vi "Read Buffer Statistic.vi"(7 "Statistic (0:Min)":i32(ring) items=["Min", "Max", "Mean", "Standard Deviation", "Peak-to-Peak"], 8 "error in (no error)":errorcluster, 10 "Instrument Model":i32(ring) items=["MODEL 6517B", "MODEL 6517A", "MODEL 6514"], 11 "VISA resource name":refnum<visa-resource-name>) -> (0 "error out":errorcluster, 2 "Statistic Value":dbl, 3 "VISA resource name out":refnum<visa-resource-name>)   [LabVIEW 2016, in "Keithley 6517.lvlib"]
doc: "Reads the specified statistic of the buffer."
uses:
  <instrlib>/Keithley 6517/Keithley 6517.lvlib
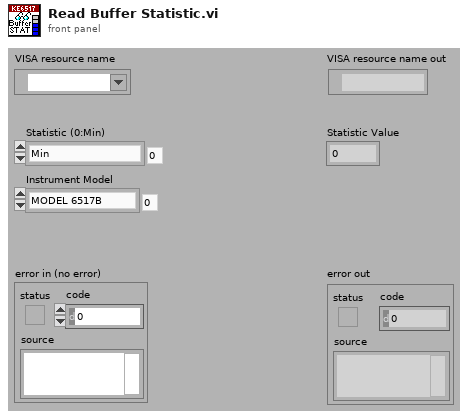
[diagram p1: front panel]
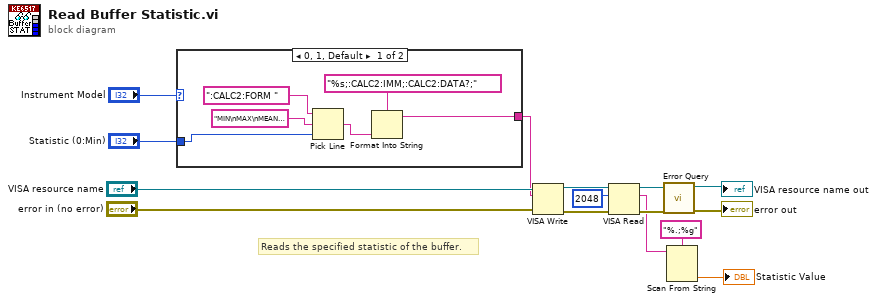
[diagram p0: block diagram]
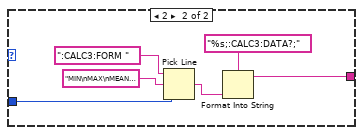
[diagram p2: hidden frame]
diagram:
  # "Reads the specified statistic of the buffer."
  n1 = case shown="0, 1, Default" "Instrument Model" {
    tunnel: "Statistic (0:Min)" -> [w16 w25]
    tunnel: [w17 w22] -> w1
    frame 0, 1, Default {
      n2 = Pick Line(string ("")=":CALC2:FORM ", multi-line string="MIN\nMAX\nMEAN\nSDEV\nPKPK", line index=w16) -> (output string=w19:string)
      n3 = Format Into String(format string="%s;:CALC2:IMM;:CALC2:DATA?;", w19) -> (resulting string=w17:string)  [unwired: 2 in, 1 out]
    }
    frame 2 {
      n4 = Pick Line(string ("")=":CALC3:FORM ", multi-line string="MIN\nMAX\nMEAN\nSDEV\nPKPK", line index=w25) -> (output string=w24:string)
      n5 = Format Into String(format string="%s;:CALC3:DATA?;", w24) -> (resulting string=w22:string)  [unwired: 2 in, 1 out]
    }
  }
  n6 = VISA Write(VISA resource name="VISA resource name", write buffer=w1, error in (no error)="error in (no error)") -> (VISA resource name out=w14:refnum<visa-resource-name>, error out=w15:errorcluster)  [unwired: 1 out]
  n7 = VISA Read(VISA resource name=w14, byte count=u32 2048, error in (no error)=w15) -> (VISA resource name out=w10:refnum<visa-resource-name>, read buffer=w6:string, error out=w11:errorcluster)  [unwired: 1 out]
  n8 = call <instrlib>:"Error Query.vi"("error in (no error)"=w11, "VISA resource name"=w10) -> ("error out"=→"error out":errorcluster, "VISA resource name out"=→"VISA resource name out":refnum<visa-resource-name>)  [unwired: 6 in, 2 out]
  n9 = Scan From String(format string="%.;%g", input string=w6) -> (output 1=→"Statistic Value":dbl)  [unwired: 3 in, 3 out]
